vi "VSI Write Bits.vi"(7 "pWriteBitStr":string, 9 "SPIIndex":i32, 10 "DevIndex":i32, 11 "DevType":i32) -> (3 "function return":i32, 5 "pWriteBitStr out":string)   [LabVIEW 2010, in "ControlSPI.lvlib"]
doc: "int WINAPI VSI_WriteBits(int DevType,int DevIndex,int SPIIndex,unsigned char *pWriteBitStr);"
uses:
  ControlSPI.lvlib
  ControlSPI/Ginkgo_Driver.dll
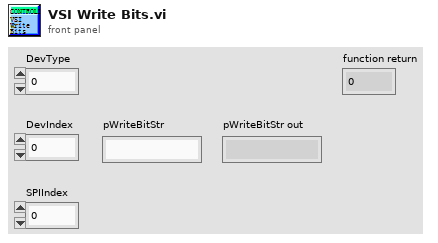
[diagram p1: front panel]
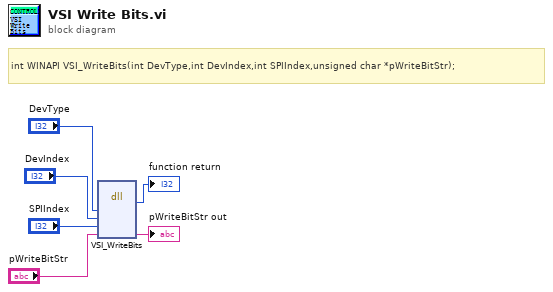
[diagram p0: block diagram]
diagram:
  # "int WINAPI VSI_WriteBits(int DevType,int DevIndex,int SPIIndex,unsigned char *pWriteBitStr);"
  n1 = dll-call lib="E:/Project/vt_ginkgo/truck/Ginkgo Driver/vs2010/Ginkgo_USB-I2C&SPI&CAN_API_v2.0.3.3/lib/labview_32bit/ControlSPI/Ginkgo_Driver.*" fn="VSI_WriteBits"("DevType"="DevType", "DevIndex"="DevIndex", "SPIIndex"="SPIIndex", "pWriteBitStr"="pWriteBitStr") -> (→"function return":i32, "pWriteBitStr"=→"pWriteBitStr out":string)  [unwired: 6 in, 2 out]
